vi "Wheel Separation to Frame Positions.vi"(11 "wheel separation":dbl) -> (0 "wheel frame angles (rad)":dbl[](array[numeric]), 1 "wheel y positions":dbl[](array[numeric]), 2 "wheel x positions":dbl[](array[numeric]), 3 "coerced wheel separation":dbl, 4 "wheel indexes":i32[](array[numeric]))   [LabVIEW 2017, in "NI_Robotics_Differential Steering Frame.lvclass"]
uses:
  <vilib>/robotics/Steering/Differential Steering Frame/NI_Robotics_Differential Steering Frame.lvclass
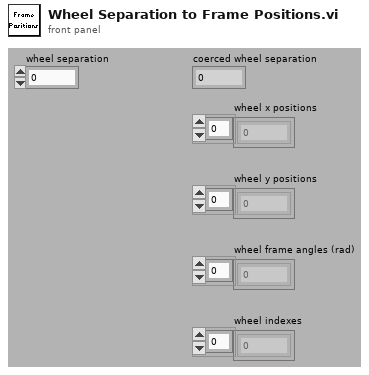
[diagram p1: front panel]
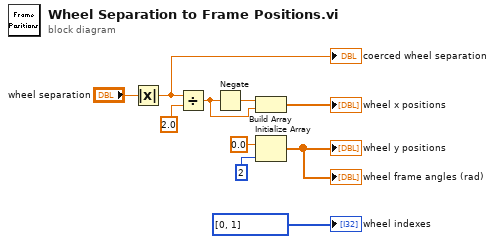
[diagram p0: block diagram]
diagram:
  n1 = Absolute Value(x="wheel separation") -> (abs(x)=w8:dbl)
  "coerced wheel separation" <- w8
  n2 = Divide(x=w8, y=2.0) -> (x/y=w7:dbl)
  n3 = Negate(x=w7) -> (-x=w6:dbl)
  n4 = Build Array(w6, w7) -> (→"wheel x positions":dbl[])
  n5 = Initialize Array(0.0 ("element"), 2 ("dimension size")) -> (→"wheel y positions" →"wheel frame angles (rad)":dbl[])
  "wheel indexes" <- i32[] [0, 1] ("wheel indexes")
